vi "EXP2.vi"() -> ()   [LabVIEW 2021]
uses:
  <vilib>/httpClient/LabVIEWHTTPClient.lvlib
panel:
  out "headers":string
  out "body":string
  in  "stop":bool
  out "error out":errorcluster
  in  "error in (no error)":errorcluster
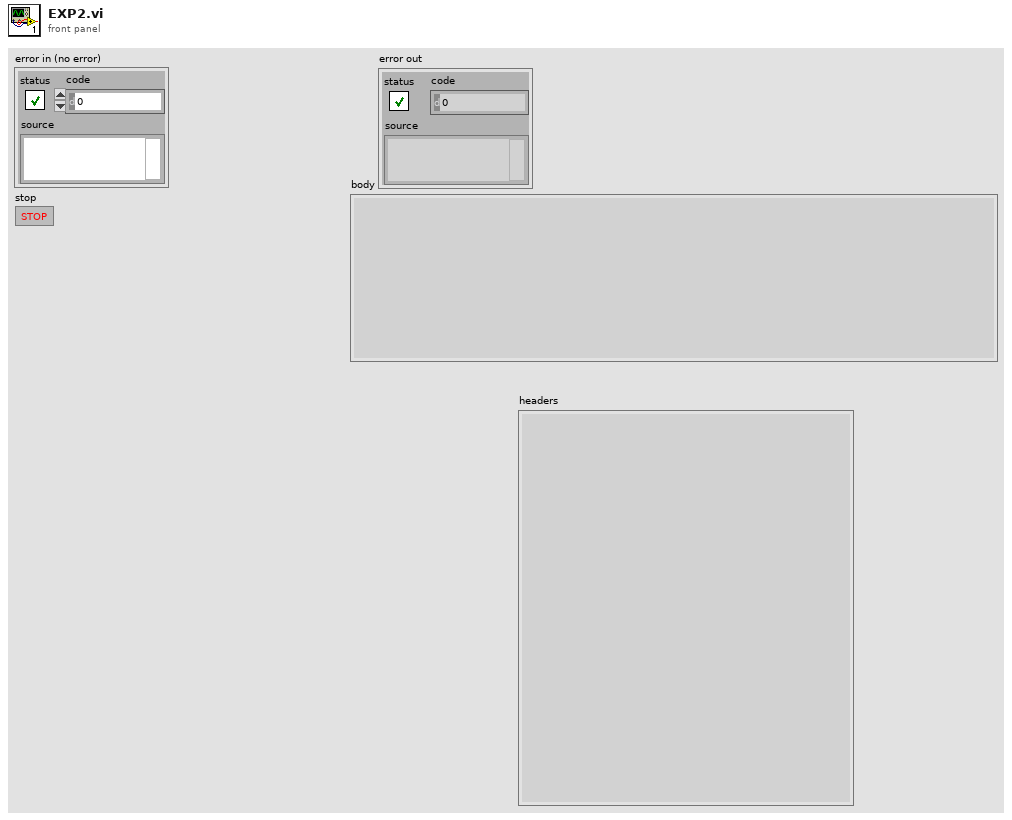
[diagram p1: front panel]
types:
  T1 = typedef "LabVIEWHTTPClient.lvlib/ClientHandle.ctl" = refnum<k1>
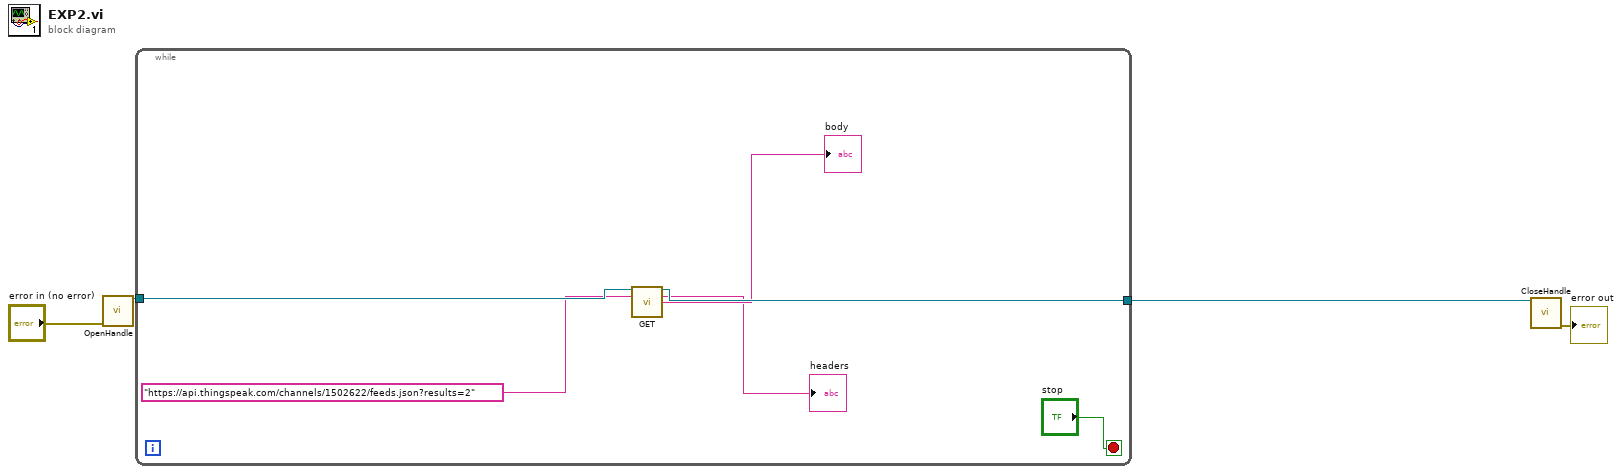
[diagram p0: block diagram]
diagram:
  n1 = call <vilib>:"OpenHandle.vi"("error in (no error)"="error in (no error)") -> ("client handle out"=w4:T1)  [unwired: 13 in, 1 out]
  n2 = while {
    tunnel: w4 -> [w10]
    tunnel: [w9] -> w3
    stop <- "stop" stop-if-true
    n3 = call <vilib>:"GET.vi"("client handle"=w10, "url"="https://api.thingspeak.com/channels/1502622/feeds.json?results=2") -> ("client handle out"=w9:T1, "headers"=→"headers":string, "body"=→"body":string)  [unwired: 10 in, 1 out]
  }
  n4 = call <vilib>:"CloseHandle.vi"("client handle"=w3) -> ("error out"=→"error out":errorcluster)  [unwired: 14 in]
